vi "UDP Send and Receive.vi"(7 "timeout ms (100)":i32=100, 8 "error in (no error)":errorcluster, 9 "Data":string, 10 "IP":string, 11 "connection ID in":refnum<k16>) -> (0 "error out":errorcluster, 1 "Received Data":T1, 2 "ACK/NACK":T2, 3 "connection ID out":refnum<k16>)   [LabVIEW 2016, in "SMD-7615.lvlib" / "eSCL.lvlib"]
uses:
  eSCL.lvlib
  UDP ACK NACK.ctl
  UDP Received Data.ctl
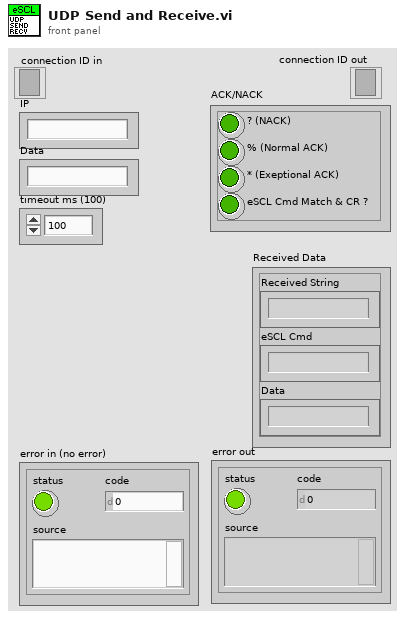
[diagram p1: front panel]
types:
  T1 = typedef "SMD-7615.lvlib/eSCL.lvlib/UDP Received Data.ctl" = cluster{"Received String":string, "eSCL Cmd":string, "Data":string}
  T2 = typedef "SMD-7615.lvlib/eSCL.lvlib/UDP ACK NACK.ctl" = cluster{"? (NACK)":bool, "% (Normal ACK)":bool, "* (Exeptional ACK)":bool, "eSCL Cmd Match & CR ?":bool}
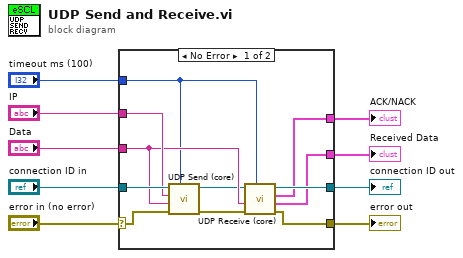
[diagram p0: block diagram]
diagram:
  n1 = case shown="No Error" "error in (no error)" {
    selector: "error in (no error)" -> [w18 w21]
    tunnel: "connection ID in" -> [w20 w22]
    tunnel: [w13 w22] -> w7
    tunnel: [w12 w21] -> w6
    tunnel: "timeout ms (100)" -> [w14 _]
    tunnel: "IP" -> [w19 _]
    tunnel: "Data" -> [w17 _]
    tunnel: [w11 _] -> w2
    tunnel: [w10 _] -> w1
    frame No Error {
      n2 = call "UDP Send (core).vi"("timeout ms (100)"=w14, "error in (no error)"=w18, "Data"=w17, "IP"=w19, "connection ID in"=w20) -> ("error out"=w15:errorcluster, "connection ID out"=w16:refnum<k16>)  [unwired: 5 in]
      n3 = call "UDP Receive (core).vi"("timeout ms (100)"=w14, "error in (no error)"=w15, "eSCL Cmd (send)"=w17, "connection ID in"=w16) -> ("error out"=w12:errorcluster, "Received Data"=w11:T1, "ACK/NACK"=w10:T2, "connection ID out"=w13:refnum<k16>)  [unwired: 4 in]
    }
    frame Error {
    }
  }
  "connection ID out" <- w7
  "error out" <- w6
  "ACK/NACK" <- w1
  "Received Data" <- w2
